vi "svx_SC Line Update Data.vi"(7 "shaft centerline":T1, 10 "index":i32, 11 "reference":refnum<vi>) -> ()   [LabVIEW 2017, in "SVX SC Line.xctl"]
uses:
  <vilib>/addons/_XControls/Shaft Centerline/SVX SC Line.xctl
  <vilib>/addons/_XControls/Shaft Centerline/subVIs/svx_SC Line Data.ctl
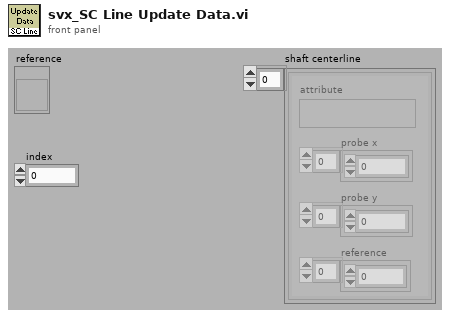
[diagram p1: front panel]
types:
  T1 = typedef "SVX SC Line.xctl/svx_SC Line Data.ctl" = cluster{"probe x":dbl[], "probe y":dbl[], "reference":dbl[], "attribute":variant}[]
  T2 = cluster{"probe x":dbl[], "probe y":dbl[], "reference":dbl[], "attribute":variant}
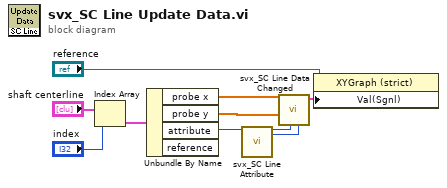
[diagram p0: block diagram]
diagram:
  n1 = Index Array(array="shaft centerline", index="index") -> (element=w2:T2)
  n2 = Unbundle By Name(w2) -> ("probe x"=w10:dbl[], "probe y"=w8:dbl[], "attribute"=w9:variant)  [unwired: 1 out]
  n3 = call <vilib>:"svx_SC Line Attribute.vi"("attribute"=w9) -> ("probe angle X"=w5:u32, "probe angle Y"=w4:u32)  [unwired: 14 in, 3 out]
  n4 = call <vilib>:"svx_SC Line Data Changed.vi"("probe angles Y"=w4, "probe angles X"=w5, "DC Y"=w8, "DC X"=w10) -> ("SC Line Data"=w7:cluster{"x":dbl[], "y":dbl[]})  [unwired: 6 in, 1 out]
  n5 = property on="Property Node" class="XYGraph (strict)"(reference="reference", "Val(Sgnl)"=w7) -> ()  [unwired: 1 in, 2 out]
